vi "FirstOrderLowpassFilter.vi"(1 "Tf":dbl, 2 "Ts":dbl, 3 "u":dbl) -> (0 "y":dbl)   [LabVIEW 2019]
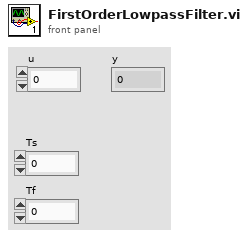
[diagram p1: front panel]
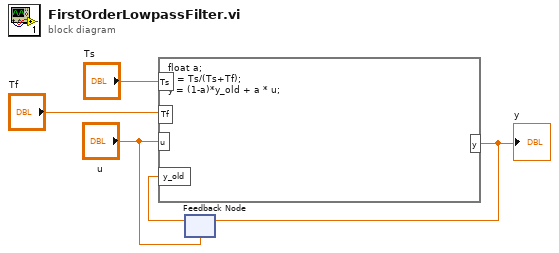
[diagram p0: block diagram]
diagram:
  n1 = feedback #1("u") -> (w4:dbl)
  n2 = formula code="float a;\na = Ts/(Ts+Tf);\ny = (1-a)*y_old + a * u;"("y_old"=w4, "u"="u", "Ts"="Ts", "Tf"="Tf") -> ("y"=w3:dbl)
  "y" <- w3
  n3 = feedback-in #1(w3) -> ()
